vi "Get_Settings_Item.vi"(8 "error in (no error)":errorcluster, 11 "IB_Settings_Item in":refnum<class "IB_Settings_Item.lvclass">) -> (0 "error out":errorcluster, 2 "data":T1, 3 "IB_Settings_Item out":refnum<class "IB_Settings_Item.lvclass">)   [LabVIEW 2020, in "IB_Settings_Item.lvclass"]
uses:
  <vilib>/AppBuilder/IB_Classes/Settings_Item/IB_Settings_Item.lvclass
  <vilib>/AppBuilder/IB_Classes/Settings_Item/IB_Settings_Item.lvclass/IB_Settings_Item.ctl
  <vilib>/AppBuilder/IB_Classes/Settings_Item/IB_Settings_Item.ctl
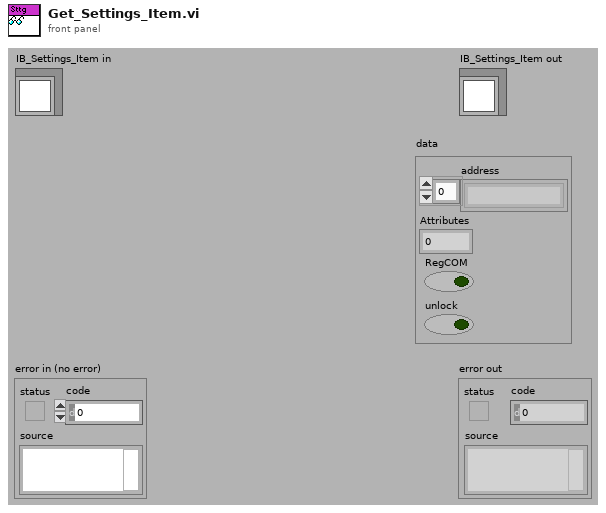
[diagram p1: front panel]
types:
  T1 = typedef "IB_Settings_Item.ctl" = cluster{"address":string[], "Attributes":i16, "RegCOM":bool, "unlock":bool}
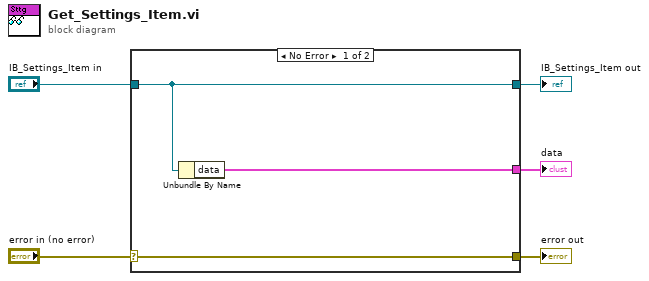
[diagram p0: block diagram]
diagram:
  n1 = case shown="No Error" "error in (no error)" {
    selector: "error in (no error)" -> [w8 w9]
    tunnel: [w8 w9] -> w4
    tunnel: [w7 w10] -> w2
    tunnel: "IB_Settings_Item in" -> [w7 w10]
    tunnel: [w6 _] -> w1
    frame No Error {
      n2 = Unbundle By Name(w7) -> ("data"=w6:T1)
    }
    frame Error {
    }
  }
  "error out" <- w4
  "IB_Settings_Item out" <- w2
  "data" <- w1
